vi "Path 1D to Data Type.vi"(8 "error in (no error)":errorcluster, 11 "Path 1D":path[](array[path])) -> (0 "error out":errorcluster, 3 "Path 1D out":refnum<class "Path 1D.lvclass">)   [LabVIEW 2017, in "Path 1D.lvclass"]
uses:
  <vilib>/gpm_packages/@cs/data-type-serializer/source/Path 1D/Path 1D.lvclass
  <vilib>/gpm_packages/@cs/data-type-serializer/source/Path 1D/Path 1D.lvclass/Path 1D.ctl
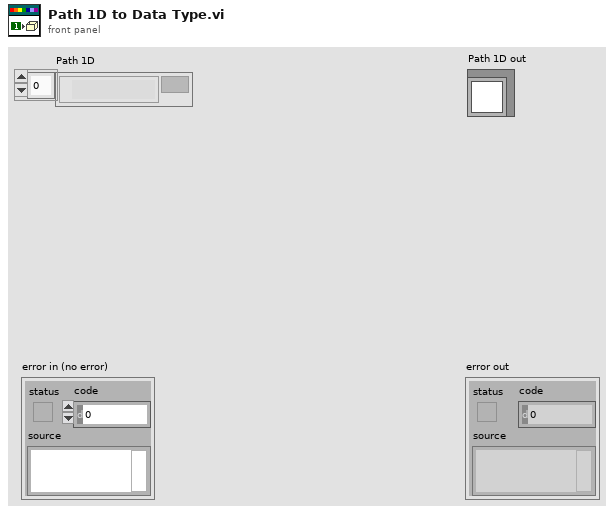
[diagram p1: front panel]
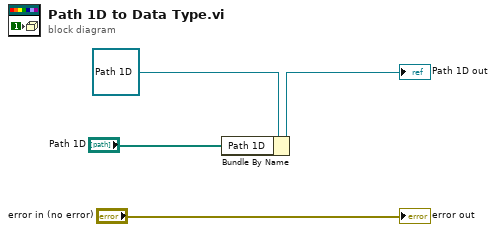
[diagram p0: block diagram]
diagram:
  n1 = Bundle By Name(cluster=refnum<class "Path 1D.lvclass"> refnum ("Boolean in"), "Path 1D"="Path 1D") -> (→"Path 1D out":refnum<class "Path 1D.lvclass">)
  "error out" <- "error in (no error)"
